vi "DataReceiverTemp.vi"() -> ()   [LabVIEW 2010]
doc: "This VI in conjunction with Target Fullness.vi demonstrates how to use network streams properties to determine how effectively data is being delivered through the network stream before it becomes congested and has to block before accepting new data. Setting the writer wait time smaller than the reader wait time will cause the reader and writer to gradually fill up. In this situation, the reader is the bottleneck of the transfer. Setting the reader wait time smaller than the writer wait time will cause the reader and writer to gradually empty. In this situation, the writer is the bottleneck of the transfer.\n\n<B>Note:</B> Requires Target Fullnes.vi located in the same directory as this VI."
uses:
  Program Files/National Instruments/LabVIEW 2010/resource/objmgr/ni.dex.rc
panel:
  out "size(s) 2":i32
  out "size(s)":i32[](array[numeric])
  out "Numeric":i32
  out "Waveform Chart":waveform(dbl)[](graph)
  in  "SamplingRate":refnum<k21>
  in  "ChannelNames":refnum<k21>="ni.var.psp://at-s1no1/AcquisitionVariables/ChannelNames"
  in  "Target IP Address":string="10.21.16.15"
  in  "Scale":dbl=1.6934e-10
  in  "Spacing":dbl=0.002
  out "error out":errorcluster
  in  "Reader Wait Time":u32=25
  in  "stop":bool
  out "Elements in Reader":i32(slide) scale=0.0..100.0
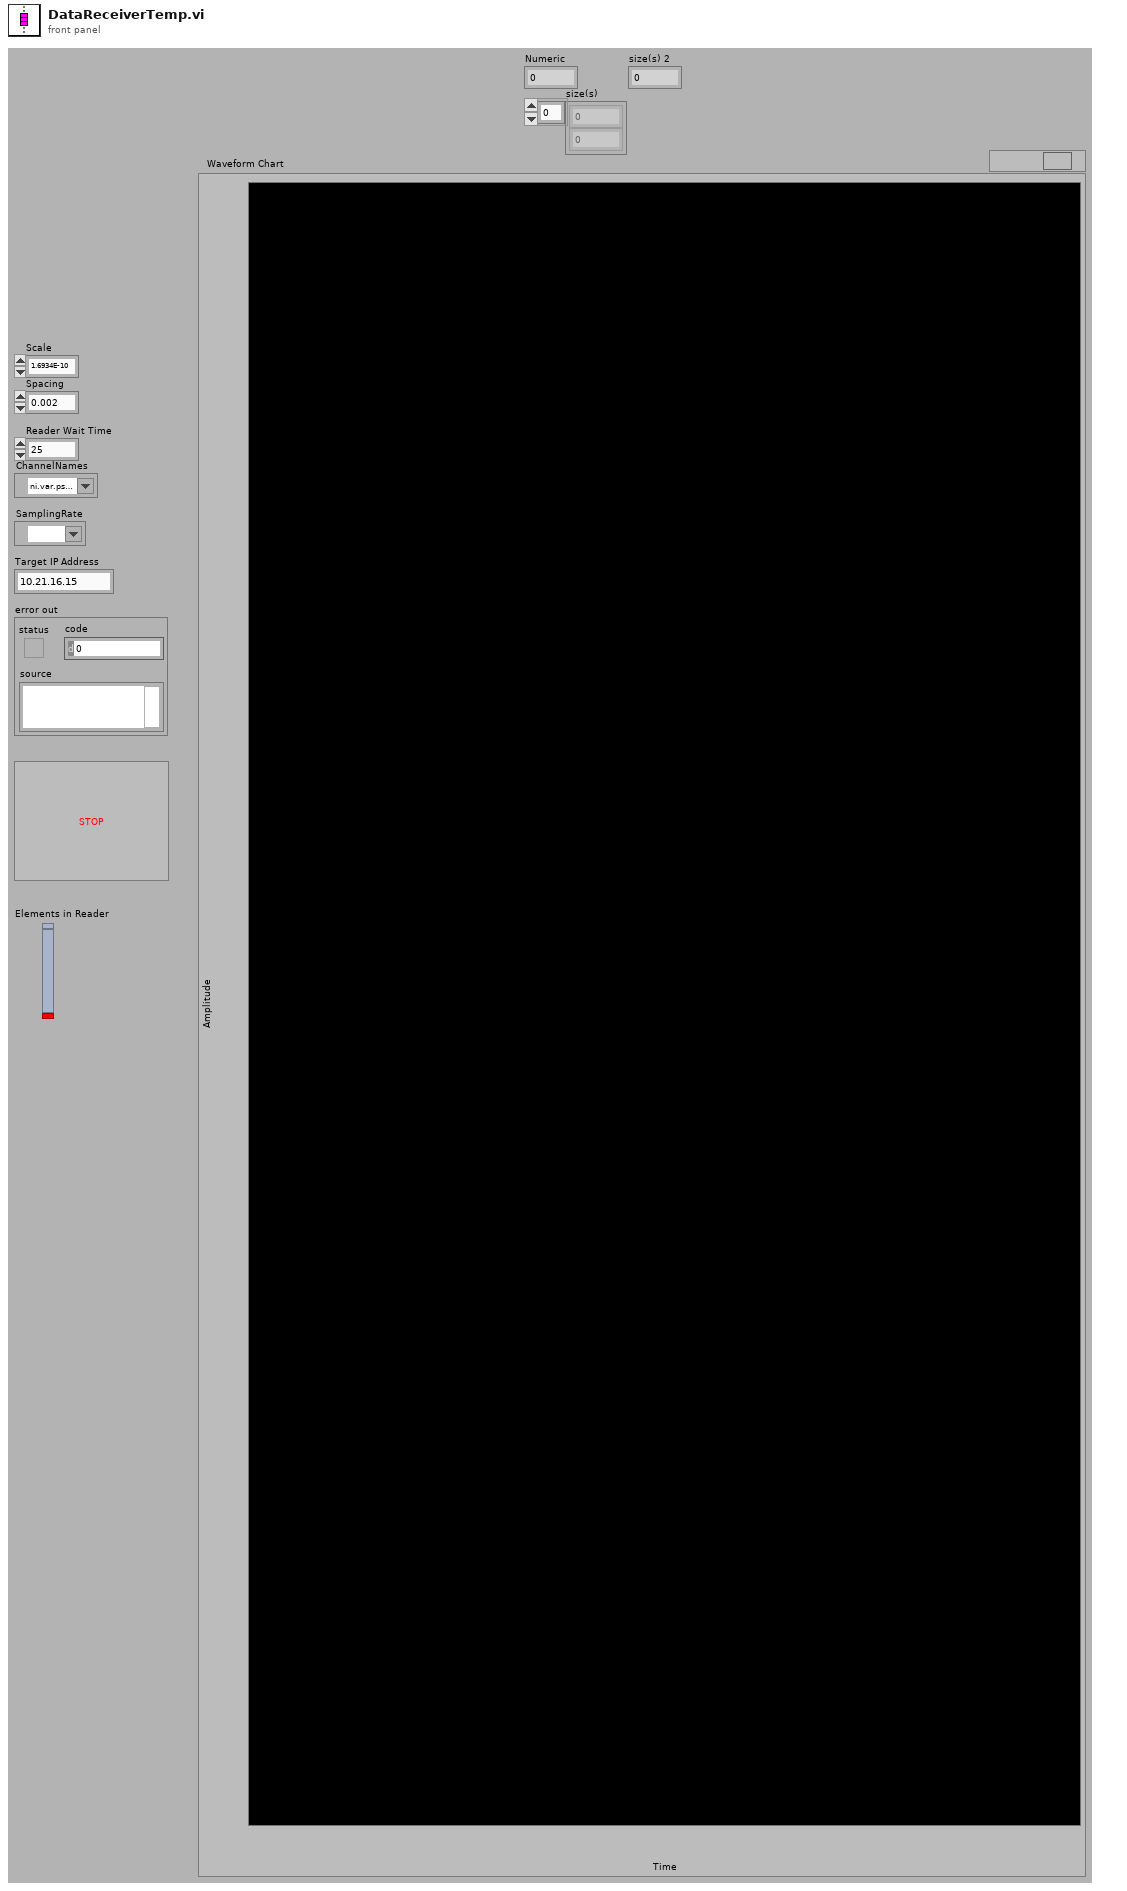
[diagram p1: front panel]
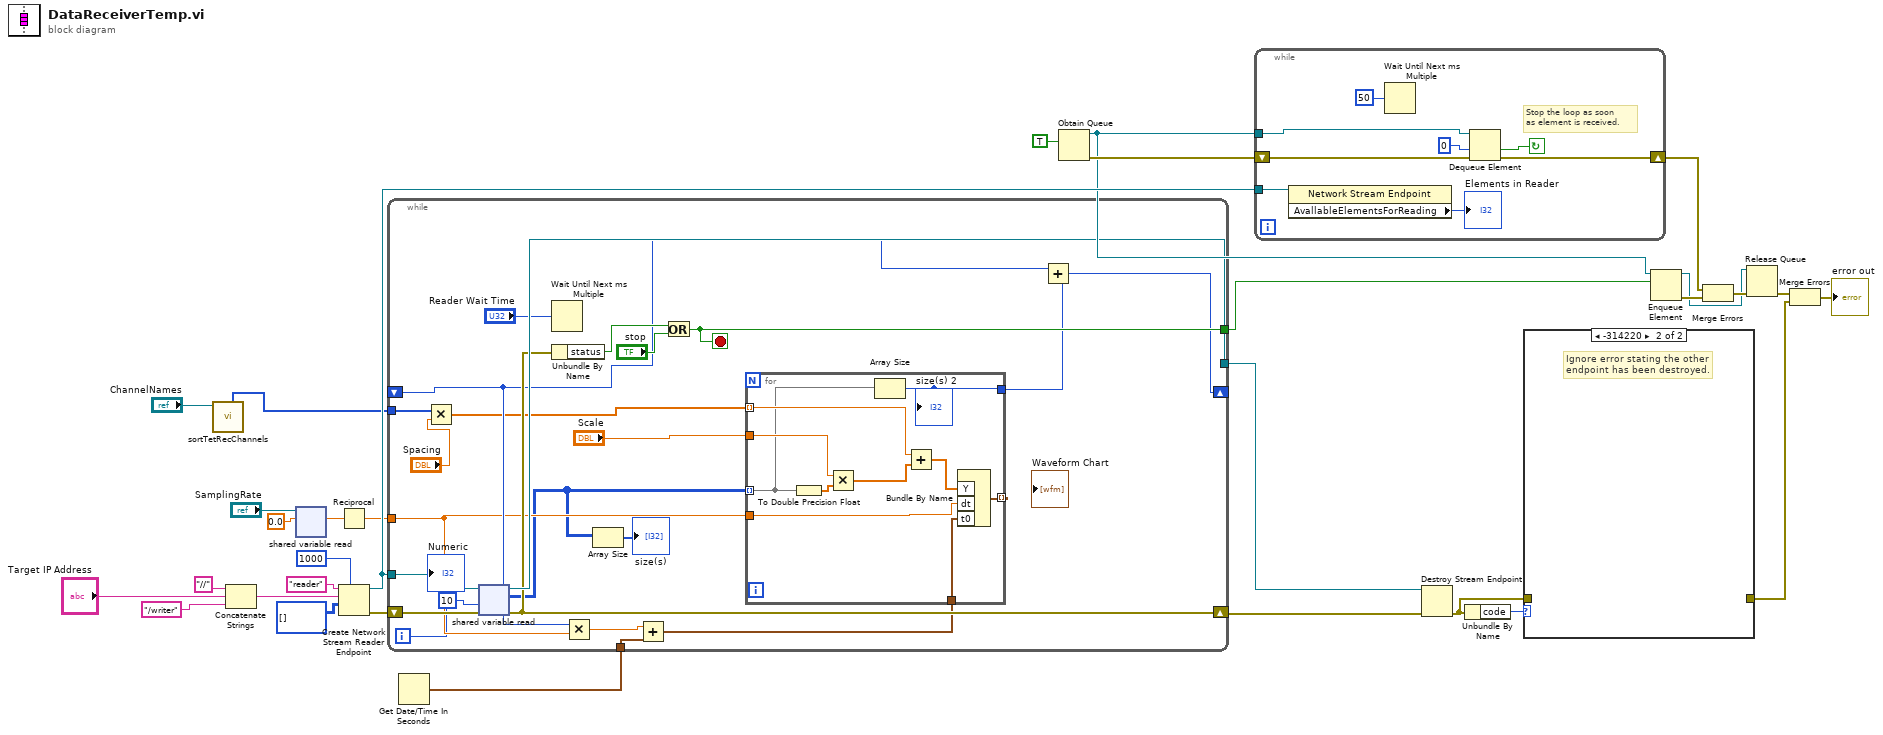
[diagram p0: block diagram]
diagram:
  n1 = call "sortTetRecChannels.vi"("shared variable refnum in"="ChannelNames") -> ("reorderedChanNums"=w1:i32[])  [unwired: 4 in, 6 out]
  n2 = Concatenate Strings("//" ("reader url"), "Target IP Address", "/writer" ("string")) -> (w8:string)
  n3 = shared-variable-read("SamplingRate", 0.0) -> (w4:dbl)  [unwired: 1 in, 3 out]
  n4 = Reciprocal(x=w4) -> (1/x=w2:dbl)
  n5 = Create Network Stream Reader Endpoint(7:1000 ("reader buffer size"), 9:i32[][] [], 10:w8, 11:"reader" ("writer name")) -> (0:w30:errorcluster, 3:w27:refnum<k21>)  [unwired: 2 in]
  n6 = Get Date/Time In Seconds() -> (seconds since 1Jan1904=w3:timestamp)
  n7 = while {
    tunnel: w27 -> [w53]
    tunnel: [w52] -> w29
    shift-right: [w47] -> w28
    shift-left: w30 -> [w54]
    tunnel: [w46] -> w16
    tunnel: w1 -> [w36]
    tunnel: w3 -> [w40]
    tunnel: w2 -> [w41]
    shift-right: [w44] -> _
    shift-left: _ -> [w42]
    i -> [w34]
    stop <- w46 stop-if-true
    n8 = Multiply(x=w36, y="Spacing") -> (x*y=w37:dbl[])
    n9 = shared-variable-read(w53, w54, 10 ("timeout in ms (-1)")) -> (w52:refnum<k21>, w47:errorcluster, w33:i32[][])  [unwired: 1 out]
    n10 = Wait Until Next ms Multiple(millisecond multiple="Reader Wait Time") -> ()  [unwired: 1 out]
    n11 = Unbundle By Name(w47) -> ("status"=w48:bool)
    n12 = Multiply(x=w42, y=w41) -> (x*y=w39:dbl)
    n13 = Array Size(array=w33) -> (size(s)=→"size(s)":i32[])
    n14 = Add(x=w39, y=w40) -> (x+y=w38:timestamp)
    n15 = Or(x=w48, y="stop") -> (x .or. y?=w46:bool)
    n16 = for {
      tunnel: w33 -> [w57] mode=indexing
      tunnel: [w64] -> _ mode=indexing
      tunnel: w37 -> [w63] mode=indexing
      tunnel: "Scale" -> [w61]
      tunnel: w41 -> [w58]
      tunnel: [w56] -> w43
      tunnel: w38 -> [w55]
      n17 = To Double Precision Float(number=w57) -> (double precision float=w62:dbl[])
      n18 = Multiply(x=w61, y=w62) -> (x*y=w60:dbl[])
      n19 = Array Size(array=w57) -> (size(s)=w56:i32)
      "size(s) 2" <- w56
      n20 = Add(x=w63, y=w60) -> (x+y=w59:dbl[])
      n21 = Bundle By Name("Y"=w59, "dt"=w58, "t0"=w55) -> (w64:waveform(dbl))  [unwired: 1 in]
    }
    n22 = Add(x=w42, y=w43) -> (x+y=w44:i32)
    "Numeric" <- w34
  }
  n23 = Obtain Queue(element data type=TRUE ("stop")) -> (queue out=w19:refnum<queue>, error out=w24:errorcluster)  [unwired: 4 in, 1 out]
  n24 = while {
    tunnel: w27 -> [w72]
    tunnel: w19 -> [w69]
    shift-right: [w67] -> w26
    shift-left: w24 -> [w66]
    stop <- w65 continue-if-true
    # "Stop the loop as soon \nas element is received."
    n25 = property class="Network Stream Endpoint"(reference=w72) -> ("AvallableElementsForReading"=→"Elements in Reader":i32)  [unwired: 1 in, 2 out]
    n26 = Wait Until Next ms Multiple(millisecond multiple=u32 50 ("milliseconds to wait")) -> ()  [unwired: 1 out]
    n27 = Dequeue Element(queue=w69, timeout in ms (-1)=0, error in (no error)=w66) -> (timed out?=w65:bool, error out=w67:errorcluster)  [unwired: 2 out]
  }
  n28 = Destroy Stream Endpoint(8:w28, 11:w29) -> (0:w17:errorcluster)
  n29 = Unbundle By Name(w17) -> ("code"=w18:i32)
  n30 = case shown="-314220" w18 {
    tunnel: w17 -> [w73 _]
    tunnel: [w73 _] -> w15
    frame 0, Default {
    }
    frame -314220 {
      # "Ignore error stating the other\nendpoint has been destroyed."
    }
  }
  n31 = Enqueue Element(queue=w19, element=w16) -> (queue out=w20:refnum<queue>, error out=w21:errorcluster)  [unwired: 2 in, 1 out]
  n32 = Merge Errors(w26, w21) -> (w23:errorcluster)
  n33 = Release Queue(queue=w20, error in (no error)=w23) -> (error out=w14:errorcluster)  [unwired: 1 in, 2 out]
  n34 = Merge Errors(w14, w15) -> (→"error out":errorcluster)
